vi "WAPIAerReadStatus-Axis.vi"(9 "error in (no error)":errorcluster) -> (0 "Axis/Plane/Queue status":T1, 6 "error out":errorcluster)   [LabVIEW 2009]
uses:
  win50032.dll
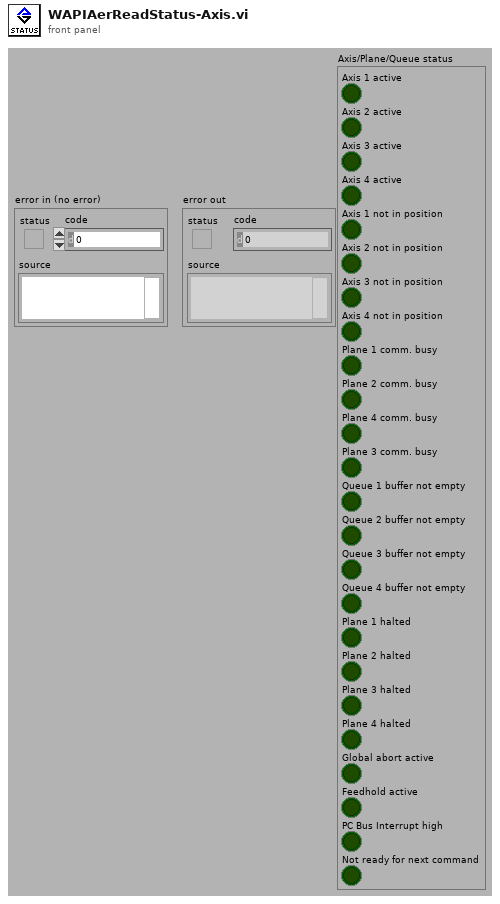
[diagram p1: front panel]
types:
  T1 = cluster{"Axis 1 active":bool, "Axis 2 active":bool, "Axis 3 active":bool, "Axis 4 active":bool, "Axis 1 not in position":bool, "Axis 2 not in position":bool, "Axis 3 not in position":bool, "Axis 4 not in position":bool, "Plane 1 comm. busy":bool, "Plane 2 comm. busy":bool, "Plane 4 comm. busy":bool, "Plane 3 comm. busy":bool, "Queue 1 buffer not empty":bool, "Queue 2 buffer not empty":bool, "Queue 3 buffer not empty":bool, "Queue 4 buffer not empty":bool, "Plane 1 halted":bool, "Plane 2 halted":bool, "Plane 3 halted":bool, "Plane 4 halted":bool, "Global abort active":bool, "Feedhold active":bool, "PC Bus Interrupt high":bool, "Not ready for next command":bool}
  T2 = cluster{"Boolean array[0]":bool, "Boolean array[1]":bool, "Boolean array[2]":bool, "Boolean array[3]":bool, "Boolean array[4]":bool, "Boolean array[5]":bool, "Boolean array[6]":bool, "Boolean array[7]":bool, "Boolean array[8]":bool, "Boolean array[9]":bool, "Boolean array[10]":bool, "Boolean array[11]":bool, "Boolean array[12]":bool, "Boolean array[13]":bool, "Boolean array[14]":bool, "Boolean array[15]":bool, "Boolean array[16]":bool, "Boolean array[17]":bool, "Boolean array[18]":bool, "Boolean array[19]":bool, "Boolean array[20]":bool, "Boolean array[21]":bool, "Boolean array[22]":bool, "Boolean array[23]":bool}
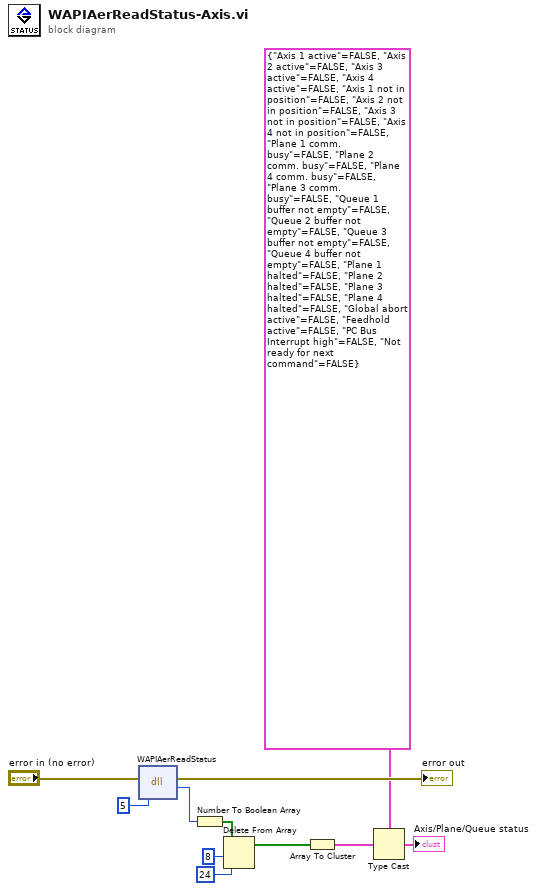
[diagram p0: block diagram]
diagram:
  n1 = dll-call lib="win50032.dll" fn="WAPIAerReadStatus"(error in="error in (no error)", "nStatus"=i16 5) -> (error out=→"error out":errorcluster, "return type"=w8:u32)  [unwired: 3 in, 1 out]
  n2 = Number To Boolean Array(number=w8) -> (Boolean array=w5:bool[])
  n3 = Delete From Array(array=w5, length=8, index=24) -> (array with subset deleted=w1:bool[])  [unwired: 1 out]
  n4 = Array To Cluster(array=w1) -> (cluster=w4:T2)
  n5 = Type Cast(type=T1 {"Axis 1 active"=FALSE, "Axis 2 active"=FALSE, "Axis 3 active"=FALSE, "Axis 4 active"=FALSE, "Axis 1 not in position"=FALSE, "Axis 2 not in position"=FALSE, "Axis 3 not in position"=FALSE, "Axis 4 not in position"=FALSE, "Plane 1 comm. busy"=FALSE, "Plane 2 comm. busy"=FALSE, "Plane 4 comm. busy"=FALSE, "Plane 3 comm. busy"=FALSE, "Queue 1 buffer not empty"=FALSE, "Queue 2 buffer not empty"=FALSE, "Queue 3 buffer not empty"=FALSE, "Queue 4 buffer not empty"=FALSE, "Plane 1 halted"=FALSE, "Plane 2 halted"=FALSE, "Plane 3 halted"=FALSE, "Plane 4 halted"=FALSE, "Global abort active"=FALSE, "Feedhold active"=FALSE, "PC Bus Interrupt high"=FALSE, "Not ready for next command"=FALSE}, x=w4) -> (*(type *) &x=→"Axis/Plane/Queue status":T1)
